vi "ScaleUp merged.vi"(8 "error in (no error)":errorcluster, 9 "left":bool=TRUE, 10 "scale":dbl=1.01, 11 "Control-Client in":refnum<class "Control-Client.lvclass">) -> (0 "error out":errorcluster, 3 "Control-Client out":refnum<class "Control-Client.lvclass">)   [LabVIEW 2019, in "Control-Client.lvclass"]
uses:
  Control-Client.lvclass
  Experiments/Experiment_merged/Experiment_merged.lvclass
  Experiments/Experiment.lvclass
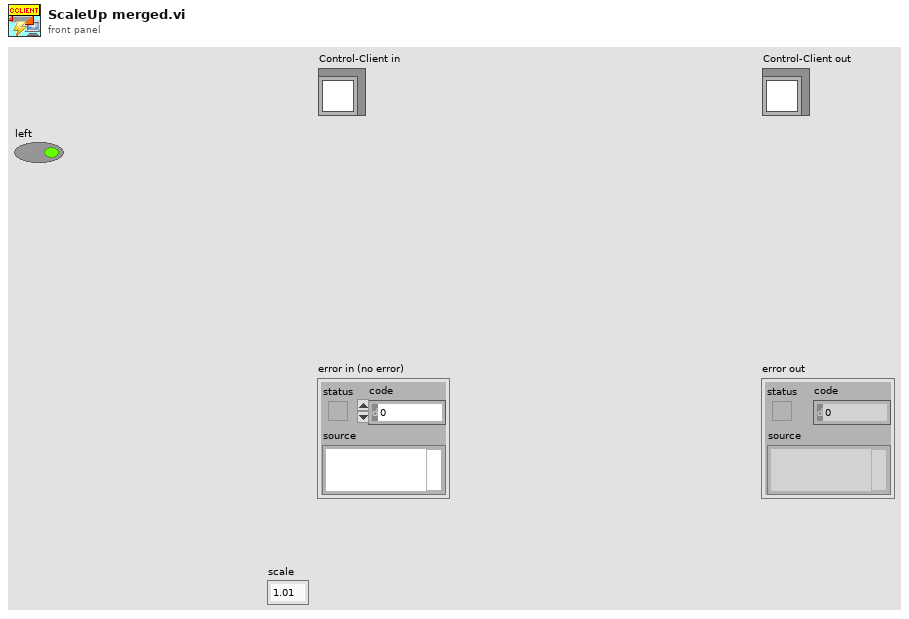
[diagram p1: front panel]
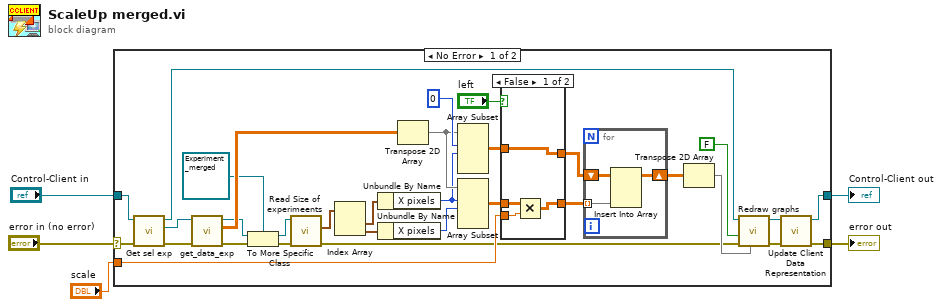
[diagram p0: block diagram]
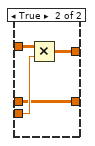
[diagram p2: hidden frame]
diagram:
  n1 = case shown="No Error" "error in (no error)" {
    selector: "error in (no error)" -> [w36 w50]
    tunnel: [w33 w50] -> w4
    tunnel: [w35 w49] -> w2
    tunnel: "Control-Client in" -> [w34 w49]
    tunnel: "scale" -> [w20 _]
    frame No Error {
      n2 = call "Get sel exp.vi"("error in (no error)"=w36, "Control-Client in"=w34) -> ("error out"=w28:errorcluster, "Sel experiment"=w37:refnum<class "Experiment.lvclass">, "Control-Client out"=w29:refnum<class "Control-Client.lvclass">)  [unwired: 7 in]
      n3 = call "get_data_exp.vi"("error in (no error)"=w28, "Experiment.lvclass in"=w37) -> ("error out"=w14:errorcluster, "Data"=w22:sgl[][], "Experiment.lvclass out"=w15:refnum<class "Experiment.lvclass">)  [unwired: 7 in]
      n4 = To More Specific Class(target class=refnum<class "Experiment_merged.lvclass"> refnum ("Experiment_merged.lvclass"), reference=w15, error in=w14) -> (specific class reference=w12:refnum<class "Experiment_merged.lvclass">, error out=w13:errorcluster)
      n5 = call-dynamic "Read Size of experimeents.vi"("error in (no error)"=w13, "Experiment_merged in"=w12) -> ("error out"=w11:errorcluster, "Size of experimeents"=w10:cluster{"X pixels":i32, "Y pixels":i32}[])  [unwired: 7 in, 1 out]
      n6 = Index Array(array=w10) -> (element #1=w9:cluster{"X pixels":i32, "Y pixels":i32}, element #2=w8:cluster{"X pixels":i32, "Y pixels":i32})  [unwired: 2 in]
      n7 = Unbundle By Name(w9) -> ("X pixels"=w7:i32)
      n8 = Unbundle By Name(w8) -> ("X pixels"=w6:i32)
      n9 = Transpose 2D Array(2D array=w22) -> (transposed array=w18:sgl[][])
      n10 = Array Subset(array=w18, index (row)=0 ("index"), length (row)=w7) -> (w25:sgl[][])  [unwired: 2 in]
      n11 = Array Subset(array=w18, index (row)=w7, length (row)=w6) -> (w26:sgl[][])  [unwired: 2 in]
      n12 = case shown="False" "left" {
        tunnel: w20 -> [w43 w48]
        tunnel: w26 -> [w44 w45]
        tunnel: w25 -> [w41 w47]
        tunnel: [w41 w46] -> w24
        tunnel: [w42 w45] -> w23
        frame False {
          n13 = Multiply(x=w44, y=w43) -> (x*y=w42:dbl[][])
        }
        frame True {
          n14 = Multiply(x=w47, y=w48) -> (x*y=w46:dbl[][])
        }
      }
      n15 = for {
        shift-right: [w39] -> w21
        shift-left: w24 -> [w40]
        tunnel: w23 -> [w38] mode=indexing
        n16 = Insert Into Array(array=w40, new element=w38) -> (w39:dbl[][])  [unwired: 2 in]
      }
      n17 = Transpose 2D Array(2D array=w21) -> (transposed array=w17:dbl[][])
      n18 = call "Redraw graphs.vi"("Data"=w17, "error in (no error)"=w11, "Selected exp"=FALSE, "Control-Client in"=w29) -> ("error out"=w32:errorcluster, "Control-Client out"=w31:refnum<class "Control-Client.lvclass">)  [unwired: 6 in]
      n19 = call "Update Client Data Representation.vi"("error in (no error)"=w32, "Control-Client in"=w31) -> ("error out"=w33:errorcluster, "Control-Client out"=w35:refnum<class "Control-Client.lvclass">)  [unwired: 8 in]
    }
    frame Error {
    }
  }
  "error out" <- w4
  "Control-Client out" <- w2
